vi "thrower Controller.vi"(8 "error in":errorcluster) -> ()   [LabVIEW 2020]
doc: "This VI executes continuously carrying out the current operation and responding to updates or new operations. It will often contain the timing or control code that is difficult to place directly in TeleOp. This VI generally opens all sensors and motors and isolates the rest of the robot code from knowing how the operations are carried out."
uses:
  <vilib>/Rock Robotics/WPI/Framework/Completion Status.ctl
  thrower Setpoints.ctl
  thrower Operations.ctl
  <vilib>/Rock Robotics/SystemInterfaces/DIO/FPGA_DIOPWMChannel.ctl
  <vilib>/Rock Robotics/SystemInterfaces/DIO/FPGA_DIOChannel.ctl
  <vilib>/Rock Robotics/WPI/ThirdParty/Phoenix-LabVIEW/Motor Controller/Controls/CTRE_Phoenix_MotorControl_ControlMode.ctl
  <vilib>/Rock Robotics/WPI/ThirdParty/REV Robotics/REVLib/Typedef/Spark MAX Control Type.ctl
  <vilib>/Rock Robotics/Network Tables/NT Write Boolean.vi
panel:
  in  "Interactive Values":T1
  out "Current\nCmd":string
  in  "Buttons":cluster{"Execute Cmd":bool, "Abort Cmd":bool}
  out "Command Timing":cluster{"Start Time (ms)":u32, "Iterations":i32}
  out "Status":T3
  # "Tip: It may be helpful to observe inputs and sensor values.\nYou may also want to display tuning or debugging controls."
  # "Interactive Command: You may fill in the settings for a command\nand schedule it with the Execute button. You can observe and abort\nany command while fine tuning the code for the controller."
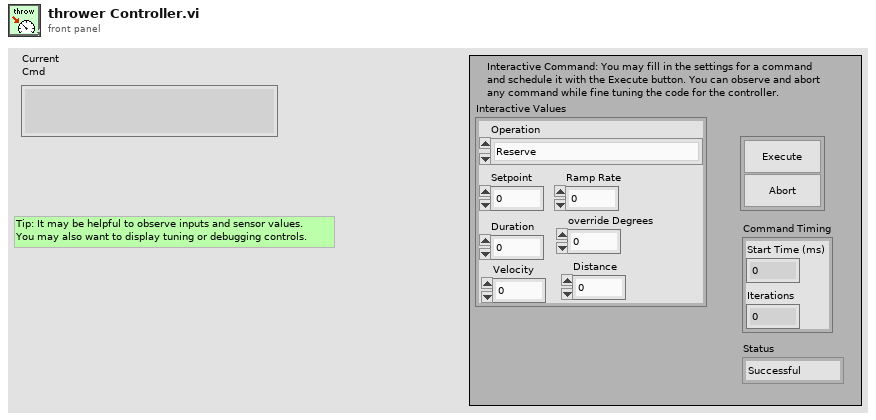
[diagram p1: front panel]
types:
  T1 = typedef "thrower Setpoints.ctl" = cluster{"Operation":T2, "Setpoint":dbl, "Duration":dbl, "Ramp Rate":dbl, "override Degrees":dbl, "Velocity":dbl, "Distance":dbl}
  T2 = typedef "thrower Operations.ctl" = enum16{"Reserve", "Read Current", "Immediate", "feed ball", "rev up thrower", "aim servos", "resetServos", "fire ball"}
  T3 = typedef "Completion Status.ctl" = enum16{"Successful", "Aborted", "Incomplete"}
  T4 = typedef "FPGA_DIOChannel.ctl" = enum8{"DIO 0", "DIO 1", "DIO 2", "DIO 3", "DIO 4", "DIO 5", "DIO 6", "DIO 7", "DIO 8", "DIO 9", "DIO MXP 0", "DIO MXP 1", "DIO MXP 2", "DIO MXP 3", "DIO MXP 4", "DIO MXP 5", "DIO MXP 6", "DIO MXP 7", "DIO MXP 8", "DIO MXP 9", "DIO MXP 10", "DIO MXP 11", "DIO MXP 12", "DIO MXP 13", "DIO MXP 14", "DIO MXP 15", "SPI Port CS1", "SPI Port CS2", "SPI Port CS3", "SPI Port MISO", "SPI Port MOSI", "Invalid"}
  T5 = typedef "FPGA_DIOPWMChannel.ctl" = enum8{"PWM 0", "PWM 1", "PWM 2", "PWM 3", "PWM 4", "PWM 5", "PWM 6", "PWM 7", "PWM 8", "PWM 9", "PWM MXP 0", "PWM MXP 1", "PWM MXP 2", "PWM MXP 3", "PWM MXP 4", "PWM MXP 5", "PWM MXP 6", "PWM MXP 7", "PWM MXP 8", "PWM MXP 9", "Invalid"}
  T6 = typedef "WPI_MotorControlDeviceRef.ctl" = cluster{"DeviceStatus":errorcluster, "Type":T7, "PWM":cluster{"PWM Channel":T5, "DeadBand":T8}, "CAN":cluster{"Device Number":u8, "SetOutput VI Ref":variant, "GetOutput VI Ref":variant, "Enable VI Ref":variant, "Disable VI Ref":variant, "Data":variant}, "Invert":bool, "DIO PWM":cluster{"PWM \"Enable\" Channel":T5, "DIOChannel":T4, "PWM Rate":dbl}}
  T7 = typedef "WPI_MotorControlType.ctl" = enum16{"PWM", "CAN", "DIO PWM"}
  T8 = typedef "WPI_PWMDeadband.ctl" = cluster{"Name":string, "maxPositivePwm":i32, "minPositivePwm":i32, "centerPwm":i32, "maxNegativePwm":i32, "minNegativePwm":i32, "angularRange":u16}
  T9 = typedef "WPI_ServoDeviceRef.ctl" = cluster{"DeviceStatus":errorcluster, "PWM Channel":T5, "DeadBand":T8}
  T10 = typedef "WPI_DigitalInputDevRef.ctl" = cluster{"DevStatus":errorcluster, "DIO Channel":T4}
  T11 = typedef "Command Status Info.ctl" = cluster{"Name":string, "Status":T3, "notifier out":T12}
  T12 = typedef "Completion Notifier.ctl" = refnum<notifier>
  T13 = cluster{"Current Command":T1, "Command Timing":cluster{"Start Time (ms)":u32, "Iterations":i32}, "Command Arguments":cluster{"Command Info":T11, "Description":string, "Default Command":T1, "queue out":refnum<queue>, "Subsystem Name":string}}
  T14 = typedef "Spark MAX Control Type.ctl" = enum16{"Percent VBus", "Voltage", "Velocity", "Position", "Smart Motion", "Current", "Smart Velocity"}
  T15 = typedef "CTRE_Phoenix_MotorControl_ControlMode.ctl" = u16
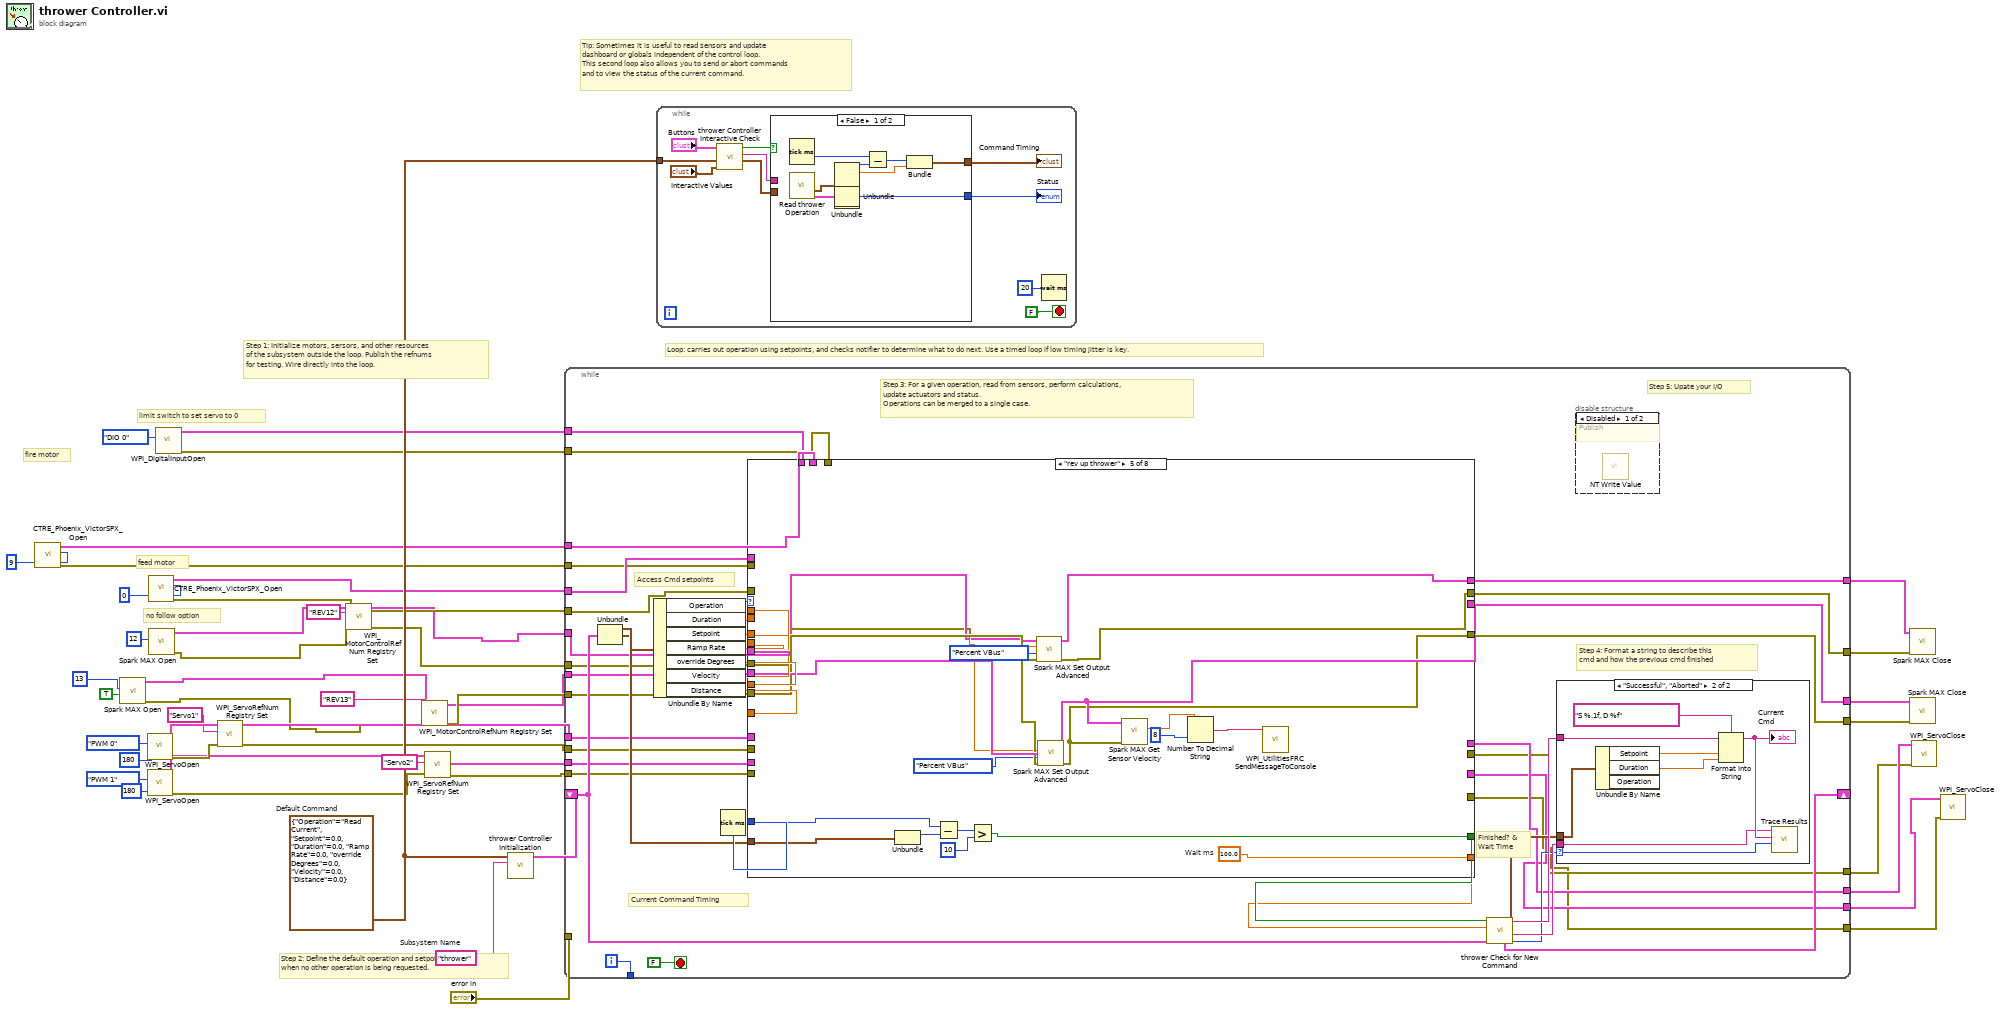
[diagram p0: block diagram]
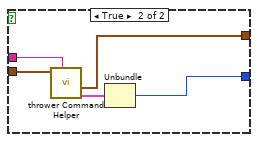
[diagram p2: hidden frame]
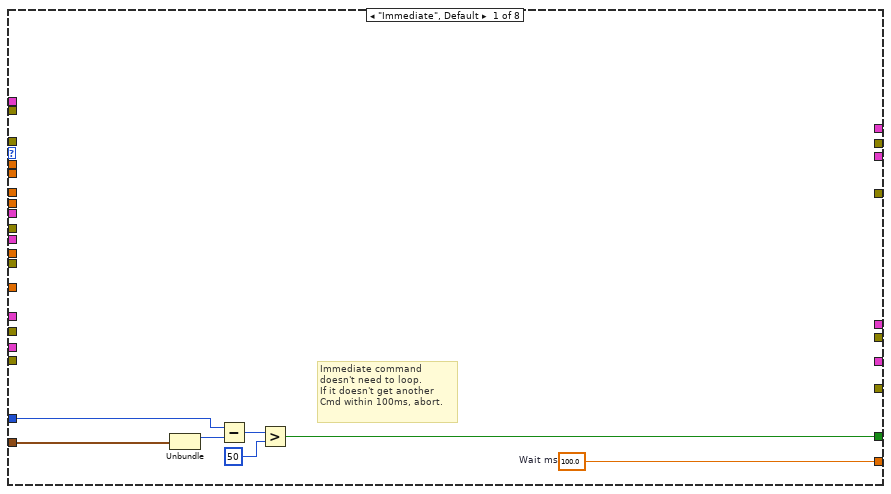
[diagram p5: hidden frame]
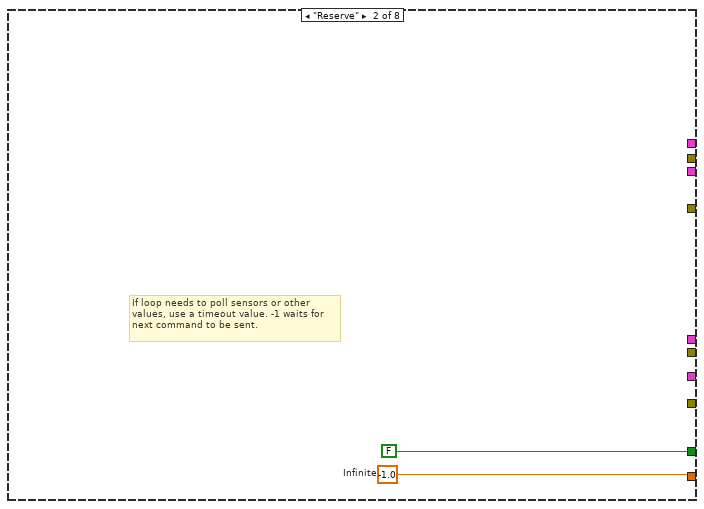
[diagram p6: hidden frame]
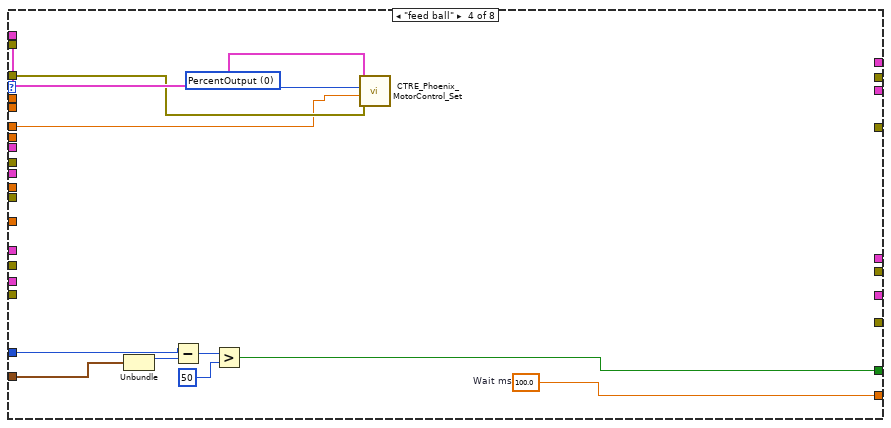
[diagram p8: hidden frame]
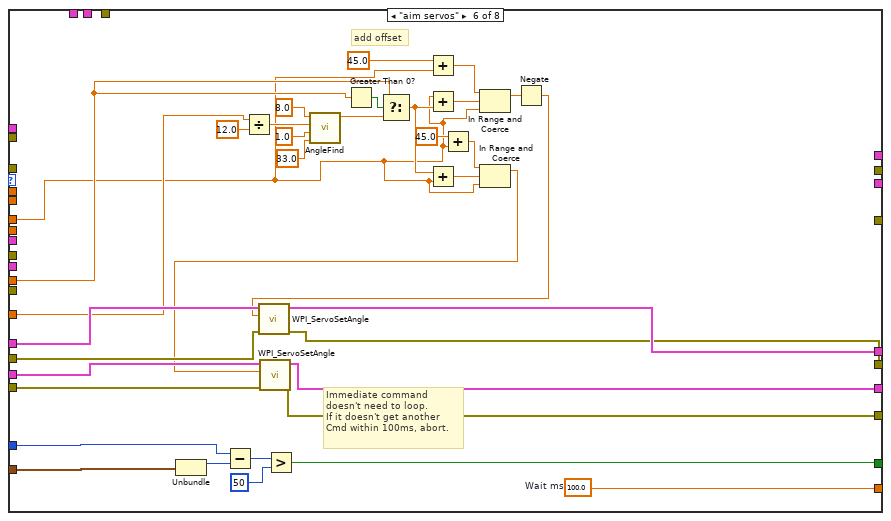
[diagram p9: hidden frame]
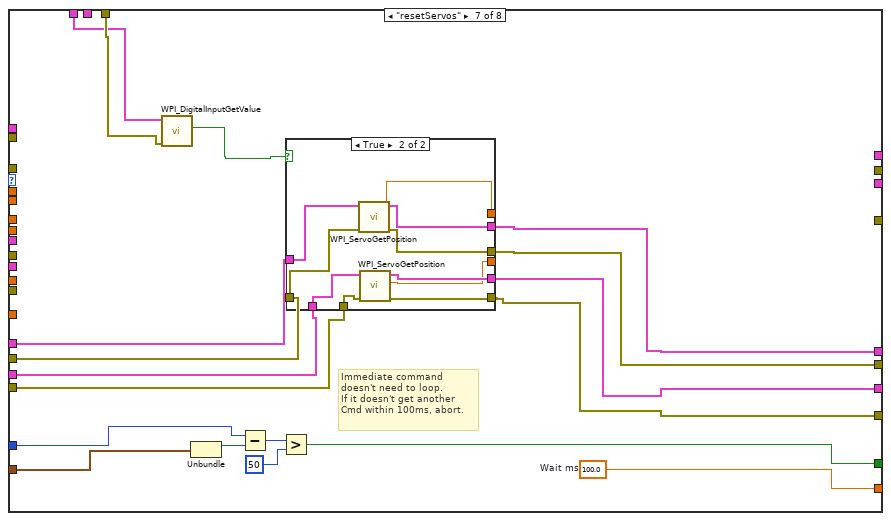
[diagram p10: hidden frame]
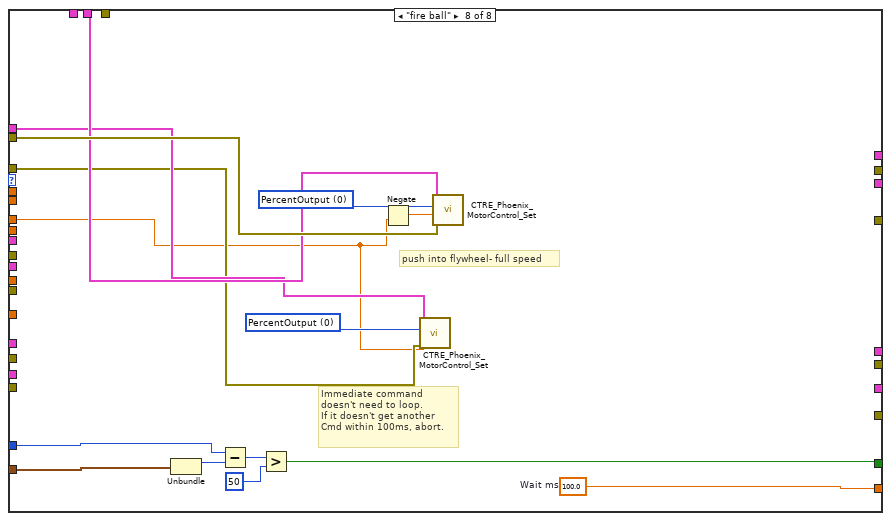
[diagram p12: hidden frame]
diagram:
  w45 = T1 {"Operation"=enum."Read Current", "Setpoint"=0.0, "Duration"=0.0, "Ramp Rate"=0.0, "override Degrees"=0.0, "Velocity"=0.0, "Distance"=0.0}  # Default Command
  w46 = "thrower"  # Subsystem Name
  # "fire motor"
  # "limit switch to set servo to 0"
  # "no follow option"
  # "feed motor"
  # "Tip: Sometimes it is useful to read sensors and update\ndashboard or globals independent of the control loop.\nThis second loop also allows you to send or abort commands\nand to view the status of the current command."
  # "Step 2: Define the default operation and setpoint --\nwhen no other operation is being requested."
  # "Step 1: Initialize motors, sersors, and other resources\nof the subsystem outside the loop. Publish the refnums\nfor testing. Wire directly into the loop."
  # "Loop: carries out operation using setpoints, and checks notifier to determine what to do next. Use a timed loop if low timing jitter is key."
  n1 = call <vilib>:"CTRE_Phoenix_VictorSPX_Open.vi"("Device Number"=u8 9) -> ("error out"=w30:errorcluster, "PhoenixMotorControlDevRef"=w31:T6)  [unwired: 9 in]
  n2 = call <vilib>:"Spark MAX Open.vi"("Invert"=TRUE, "Device Number"=u8 13) -> ("error out"=w7:errorcluster, "MotorControlDeviceRef"=w6:T6)  [unwired: 8 in]
  n3 = call <vilib>:"WPI_ServoOpen.vi"("Angular Range"=u16 180, "PWM Channel"=FPGA_DIOPWMChannel."PWM 0") -> ("error out"=w19:errorcluster, "ServoDeviceRef"=w18:T9)  [unwired: 8 in]
  n4 = call <vilib>:"WPI_ServoOpen.vi"("Angular Range"=u16 180, "PWM Channel"=FPGA_DIOPWMChannel."PWM 1") -> ("error out"=w15:errorcluster, "ServoDeviceRef"=w12:T9)  [unwired: 8 in]
  n5 = call <vilib>:"CTRE_Phoenix_VictorSPX_Open.vi"("Device Number"=u8 0) -> ("error out"=w43:errorcluster, "PhoenixMotorControlDevRef"=w44:T6)  [unwired: 9 in]
  n6 = call <vilib>:"Spark MAX Open.vi"("Device Number"=u8 12) -> ("error out"=w4:errorcluster, "MotorControlDeviceRef"=w5:T6)  [unwired: 9 in]
  n7 = call <vilib>:"WPI_DigitalInputOpen.vi"("DIO Channel"=FPGA_DIOChannel."DIO 0") -> ("error out"=w35:errorcluster, "DigitalInputDevRef"=w34:T10)  [unwired: 9 in]
  n8 = call <vilib>:"WPI_ServoRefNum Registry Set.vi"("error in (no error)"=w19, "refnum name"="Servo1", "ServoDeviceRef"=w18) -> ("error out"=w16:errorcluster, "ServoDeviceRef"=w17:T9)  [unwired: 7 in]
  n9 = call <vilib>:"WPI_MotorControlRefNum Registry Set.vi"("error in (no error)"=w4, "refnum name"="REV12", "MotorControlDevRef"=w5) -> ("error out"=w21:errorcluster, "MotorControlDevRef"=w20:T6)  [unwired: 7 in]
  n10 = call <vilib>:"WPI_MotorControlRefNum Registry Set.vi"("error in (no error)"=w7, "refnum name"="REV13", "MotorControlDevRef"=w6) -> ("error out"=w23:errorcluster, "MotorControlDevRef"=w3:T6)  [unwired: 7 in]
  n11 = call <vilib>:"WPI_ServoRefNum Registry Set.vi"("error in (no error)"=w15, "refnum name"="Servo2", "ServoDeviceRef"=w12) -> ("error out"=w14:errorcluster, "ServoDeviceRef"=w13:T9)  [unwired: 7 in]
  n12 = call "thrower Controller Initialization.vi"("Subsystem Name"=w46, "Default Command"=w45) -> ("Current Command"=w47:T13)  [unwired: 9 in]
  n13 = while {
    shift-right: [w82] -> _
    shift-left: w47 -> [w75]
    tunnel: [w89] -> _
    tunnel: "error in" -> [_]
    tunnel: w44 -> [w74]
    tunnel: w43 -> [w73]
    tunnel: w20 -> [w72]
    tunnel: w3 -> [w71]
    tunnel: w21 -> [w70]
    tunnel: w23 -> [w69]
    tunnel: w17 -> [w67]
    tunnel: w13 -> [w66]
    tunnel: w16 -> [w65]
    tunnel: w14 -> [w64]
    tunnel: [w63] -> w39
    tunnel: [w62] -> w38
    tunnel: [w61] -> w37
    tunnel: [w60] -> w36
    tunnel: w35 -> [w50]
    tunnel: w34 -> [w49]
    tunnel: w31 -> [w56]
    tunnel: w30 -> [w55]
    tunnel: [w54] -> w29
    tunnel: [w53] -> w28
    tunnel: [w52] -> w27
    tunnel: [w51] -> w26
    i -> [w89]
    stop <- FALSE stop-if-true
    # "Step 5: Upate your I/O"
    # "Step 4: Format a string to describe this\ncmd and how the previous cmd finished"
    # "Current Command Timing"
    # "Access Cmd setpoints"
    # "Finished? &\nWait Time"
    # "Step 3: For a given operation, read from sensors, perform calculations,\nupdate actuators and status.\nOperations can be merged to a single case."
    n14 = Unbundle(w75) -> ("Current Command"=w88:T1, "Command Timing"=w84:cluster{"Start Time (ms)":u32, "Iterations":i32})  [unwired: 1 out]
    n15 = Unbundle By Name(w88) -> ("Operation"=w87:T2, "Duration"=w86:dbl, "Setpoint"=w83:dbl, "Ramp Rate"=w68:dbl, "override Degrees"=w59:dbl, "Velocity"=w58:dbl, "Distance"=w57:dbl)
    n16 = Tick Count (ms)() -> (millisecond timer value=w85:u32)
    n17 = case shown="\"rev up thrower\"" w87 {
      tunnel: [w105 w107 _ w109 w137 w140 w177 w203] -> w80
      tunnel: [w99 FALSE ("ignore previous (F)") _ w110 w136 w141 w178 w204] -> w81
      tunnel: w84 -> [w101 _ _ w112 w139 w142 w179 w205]
      tunnel: w86 -> [_ _ _ _ _ _ _ _]
      tunnel: w85 -> [w100 _ _ w111 w138 w143 w180 w206]
      tunnel: w83 -> [_ _ _ w108 w131 w147 _ w210]
      tunnel: w74 -> [_ _ _ w118 _ _ _ w213]
      tunnel: w73 -> [_ _ _ w117 _ _ _ w212]
      tunnel: w72 -> [_ _ _ _ w129 _ _ _]
      tunnel: w71 -> [_ _ _ _ w135 _ _ _]
      tunnel: w70 -> [_ _ _ _ w128 _ _ _]
      tunnel: w69 -> [_ _ _ _ w134 _ _ _]
      tunnel: w68 -> [_ _ _ _ _ _ _ _]
      tunnel: w67 -> [_ _ _ _ _ w174 w191 _]
      tunnel: w66 -> [_ _ _ _ _ w173 w187 _]
      tunnel: w65 -> [_ _ _ _ _ w172 w190 _]
      tunnel: w64 -> [_ _ _ _ _ w171 w186 _]
      tunnel: [_ _ _ _ _ w170 w189 _] -> w63
      tunnel: [_ _ _ _ _ w169 w188 _] -> w62
      tunnel: [_ _ _ _ _ w168 w184 _] -> w61
      tunnel: [_ _ _ _ _ w167 w185 _] -> w60
      tunnel: w59 -> [_ _ _ _ _ w158 _ _]
      tunnel: w58 -> [_ _ _ _ _ _ _ _]
      tunnel: w57 -> [_ _ _ _ _ w157 _ _]
      tunnel: w56 -> [_ _ _ _ _ _ _ w214]
      tunnel: w55 -> [_ _ _ _ _ _ _ w215]
      tunnel: [_ _ _ _ w130 _ _ _] -> w54
      tunnel: [_ _ _ _ w127 _ _ _] -> w53
      tunnel: [_ _ _ _ w133 _ _ _] -> w52
      tunnel: [_ _ _ _ w132 _ _ _] -> w51
      tunnel: w50 -> [_ _ _ _ _ _ w176 _]
      tunnel: w49 -> [_ _ _ _ _ _ w175 _]
      frame "Immediate", Default {
        w105 = 100.0  # Wait ms
        # "Immediate command\ndoesn't need to loop.\nIf it doesn't get another\nCmd within 100ms, abort."
        n18 = Unbundle(w101) -> ("Start Time (ms)"=w104:u32)  [unwired: 1 out]
        n19 = Subtract(x=w100, y=w104) -> (x-y=w103:u32)
        n20 = Greater?(x=w103, y=u8 50 ("Left Motor")) -> (0:w99:bool)
      }
      frame "Reserve" {
        w107 = -1.0  # Infinite
        # "If loop needs to poll sensors or other\nvalues, use a timeout value. -1 waits for\nnext command to be sent."
      }
      frame "Read Current" {
      }
      frame "feed ball" {
        w109 = 100.0  # Wait ms
        w116 = T15 0 items=["PercentOutput"=0, "Position"=1, "Velocity"=2, "Current"=3, "Follower"=5, "MotionProfile"=6, "MotionMagic"=7, "MotionProfileArc"=10, "Disabled"=15] ("Control Mode")
        n21 = Unbundle(w112) -> ("Start Time (ms)"=w115:u32)  [unwired: 1 out]
        n22 = Subtract(x=w111, y=w115) -> (x-y=w114:u32)
        n23 = Greater?(x=w114, y=u8 50 ("Left Motor")) -> (0:w110:bool)
        n24 = call <vilib>:"CTRE_Phoenix_MotorControl_Set.vi"("error in (no error)"=w117, "Output"=w108, "Control Mode"=w116, "PhoenixMotorControlDevRef"=w118) -> ()  [unwired: 6 in, 2 out]
      }
      frame "rev up thrower" {
        w137 = 100.0  # Wait ms
        n25 = Unbundle(w139) -> ("Start Time (ms)"=w126:u32)  [unwired: 1 out]
        n26 = Subtract(x=w138, y=w126) -> (x-y=w125:u32)
        n27 = Greater?(x=w125, y=u8 10 ("Left Motor")) -> (0:w136:bool)
        n28 = call <vilib>:"Spark MAX Set Output Advanced.vi"("error in (no error)"=w128, "Control Mode"=Spark_MAX_Control_Type."Percent VBus", "Setpoint"=w131, "MotorControlDevRef"=w129) -> ("error out"=w127:errorcluster, "MotorControlDevRef"=w130:T6)  [unwired: 6 in]
        n29 = call <vilib>:"Spark MAX Set Output Advanced.vi"("error in (no error)"=w134, "Control Mode"=Spark_MAX_Control_Type."Percent VBus", "Setpoint"=w131, "MotorControlDevRef"=w135) -> ("error out"=w132:errorcluster, "MotorControlDevRef"=w133:T6)  [unwired: 6 in]
        n30 = call <vilib>:"Spark MAX Get Sensor Velocity.vi"("error in (no error)"=w132, "MotorControlDevRef in"=w133) -> ("Sensor Velocity"=w123:dbl)  [unwired: 6 in, 3 out]
        n31 = Number To Decimal String(number=w123, width (-)=i16 8) -> (decimal integer string=w121:string)
        n32 = call <vilib>:"WPI_UtilitiesFRC SendMessageToConsole.vi"("Message"=w121) -> ()  [unwired: 14 in, 1 out]
      }
      frame "aim servos" {
        w140 = 100.0  # Wait ms
        # "Immediate command\ndoesn't need to loop.\nIf it doesn't get another\nCmd within 100ms, abort."
        # "add offset"
        n33 = Unbundle(w142) -> ("Start Time (ms)"=w146:u32)  [unwired: 1 out]
        n34 = Subtract(x=w143, y=w146) -> (x-y=w145:u32)
        n35 = Divide(x=w157, y=12.0) -> (x/y=w161:dbl)
        n36 = Greater?(x=w145, y=u8 50 ("Left Motor")) -> (0:w141:bool)
        n37 = call "AngleFind.vi"("Speed Sent (ft)"=33.0, "Distance off Ground (ft)"=1.0, "Distance to Target (Ground Distance) (ft)"=w161, "Height of Target (ft)"=8.0) -> ("Angle (Degrees?)"=w159:dbl)  [unwired: 7 in]
        n38 = Greater Than 0?(x=w158) -> (x > 0?=w160:bool)
        n39 = Select(t=w158, s=w160, f=w159) -> (s? t:f=w156:dbl)
        n40 = Add(x=45.0, y=w147) -> (x+y=w151:dbl)
        n41 = Add(x=w147, y=w156) -> (x+y=w152:dbl)
        n42 = Add(x=w156, y=w147) -> (x+y=w153:dbl)
        n43 = Add(x=45.0, y=w147) -> (x+y=w148:dbl)
        n44 = In Range and Coerce(upper limit=w151, x=w152, lower limit=w147) -> (coerced(x)=w155:dbl)  [unwired: 1 out]
        n45 = In Range and Coerce(upper limit=w148, x=w153, lower limit=w147) -> (coerced(x)=w154:dbl)  [unwired: 1 out]
        n46 = call <vilib>:"WPI_ServoSetAngle.vi"("error in (no error)"=w171, "Angle"=w154, "ServoDeviceRef"=w173) -> ("error out"=w167:errorcluster, "ServoDeviceRef"=w168:T9)  [unwired: 7 in]
        n47 = Negate(x=w155) -> (-x=w166:dbl)
        n48 = call <vilib>:"WPI_ServoSetAngle.vi"("error in (no error)"=w172, "Angle"=w166, "ServoDeviceRef"=w174) -> ("error out"=w169:errorcluster, "ServoDeviceRef"=w170:T9)  [unwired: 7 in]
      }
      frame "resetServos" {
        w177 = 100.0  # Wait ms
        # "Immediate command\ndoesn't need to loop.\nIf it doesn't get another\nCmd within 100ms, abort."
        n49 = call <vilib>:"WPI_DigitalInputGetValue.vi"("error in (no error)"=w176, "DigitalInputDevRef"=w175) -> ("Value"=w192:bool)  [unwired: 7 in, 2 out]
        n50 = Unbundle(w179) -> ("Start Time (ms)"=w183:u32)  [unwired: 1 out]
        n51 = Subtract(x=w180, y=w183) -> (x-y=w182:u32)
        n52 = Greater?(x=w182, y=u8 50 ("Left Motor")) -> (0:w178:bool)
        n53 = case shown="True" w192 {
          tunnel: w191 -> [_ w202]
          tunnel: w190 -> [_ w201]
          tunnel: [_ w200] -> w189
          tunnel: [_ w199] -> w188
          tunnel: w187 -> [_ w198]
          tunnel: w186 -> [_ w197]
          tunnel: [_ w196] -> w185
          tunnel: [_ w195] -> w184
          tunnel: [_ w194] -> _
          tunnel: [_ w193] -> _
          frame False {
          }
          frame True {
            n54 = call <vilib>:"WPI_ServoGetPosition.vi"("error in (no error)"=w201, "ServoDeviceRef"=w202) -> ("error out"=w199:errorcluster, "Position"=w194:dbl, "ServoDeviceRef"=w200:T9)  [unwired: 7 in]
            n55 = call <vilib>:"WPI_ServoGetPosition.vi"("error in (no error)"=w197, "ServoDeviceRef"=w198) -> ("error out"=w196:errorcluster, "Position"=w193:dbl, "ServoDeviceRef"=w195:T9)  [unwired: 7 in]
          }
        }
      }
      frame "fire ball" {
        w203 = 100.0  # Wait ms
        w216 = T15 0 items=["PercentOutput"=0, "Position"=1, "Velocity"=2, "Current"=3, "Follower"=5, "MotionProfile"=6, "MotionMagic"=7, "MotionProfileArc"=10, "Disabled"=15] ("Control Mode")
        w217 = T15 0 items=["PercentOutput"=0, "Position"=1, "Velocity"=2, "Current"=3, "Follower"=5, "MotionProfile"=6, "MotionMagic"=7, "MotionProfileArc"=10, "Disabled"=15] ("Control Mode")
        # "Immediate command\ndoesn't need to loop.\nIf it doesn't get another\nCmd within 100ms, abort."
        # "push into flywheel- full speed"
        n56 = Unbundle(w205) -> ("Start Time (ms)"=w208:u32)  [unwired: 1 out]
        n57 = Subtract(x=w206, y=w208) -> (x-y=w209:u32)
        n58 = Greater?(x=w209, y=u8 50 ("Left Motor")) -> (0:w204:bool)
        n59 = Negate(x=w210) -> (-x=w211:dbl)
        n60 = call <vilib>:"CTRE_Phoenix_MotorControl_Set.vi"("error in (no error)"=w212, "Output"=w210, "Control Mode"=w216, "PhoenixMotorControlDevRef"=w213) -> ()  [unwired: 6 in, 2 out]
        n61 = call <vilib>:"CTRE_Phoenix_MotorControl_Set.vi"("error in (no error)"=w215, "Output"=w211, "Control Mode"=w217, "PhoenixMotorControlDevRef"=w214) -> ()  [unwired: 6 in, 2 out]
      }
    }
    n62 = call "thrower Check for New Command.vi"("Current Command"=w75, "Wait time (ms)"=w80, "Finished?"=w81) -> ("Completion"=w76:T3, "Subsystem Name"=w77:string, "Current Command"=w78:T1, "Initial Trace String"=w79:string, "NextCommand"=w82:T13)  [unwired: 4 in]
    n63 = case shown="\"Successful\", \"Aborted\"" w76 {
      selector: w76 -> [_ w98]
      tunnel: w79 -> [_ w94]
      tunnel: w78 -> [_ w95]
      tunnel: w77 -> [_ w91]
      frame "Incomplete", Default {
        # "Continuing current command"
      }
      frame "Successful", "Aborted" {
        # "Report and setup for next command"
        n64 = Unbundle By Name(w95) -> ("Setpoint"=w97:dbl, "Duration"=w92:dbl)  [unwired: 1 out]
        n65 = Format Into String(format string="S %.1f, D %f", initial string=w94, w97, w92) -> (resulting string=w93:string)  [unwired: 1 in, 1 out]
        "Current\nCmd" <- w93
        n66 = call <vilib>:"Trace Results.vi"("Status of previous command"=w98, "Description"=w93, "Subsystem"=w91) -> ()  [unwired: 9 in]
      }
    }
    n67 = disable-structure shown="Disabled" {
      frame Disabled {
        # "Publish"
        n68 = call-poly <vilib>:"NT Write Value.vi"() -> ()  [unwired: 11 in, 1 out]
      }
      frame Enabled {
      }
    }
  }
  n69 = while {
    tunnel: w45 -> [w218]
    stop <- FALSE stop-if-true
    n70 = call "thrower Controller Interactive Check.vi"("Interactive Command in"="Interactive Values", "Default Command"=w218, "Buttons"="Buttons") -> ("Interactive Command out"=w222:T1, "Trace String"=w223:string, "Schedule"=w224:bool)  [unwired: 6 in]
    n71 = case shown="False" w224 {
      tunnel: [w235 w240] -> w221
      tunnel: w222 -> [_ w238]
      tunnel: [w231 w236] -> w220
      tunnel: w223 -> [_ w239]
      frame False {
        n72 = Tick Count (ms)() -> (millisecond timer value=w230:u32)
        n73 = call "Read thrower Operation.vi"() -> ("Command Info"=w228:T11, "SubSystem Data"=w229:T1)  [unwired: 9 in, 1 out]
        n74 = Unbundle(w229) -> ("Operation"=w234:T2, "Setpoint"=w232:dbl)  [unwired: 5 out]
        n75 = Unbundle(w228) -> ("Status"=w235:T3)  [unwired: 2 out]
        n76 = Subtract(x=w230, y=w234) -> (x-y=w233:u32)
        n77 = Bundle(w233, "Setpoint"=w232) -> (w231:cluster{u32, "Setpoint":dbl})  [unwired: 1 in]
      }
      frame True {
        n78 = call "thrower Command Helper.vi"("Description"=w239, "SubSystem Data"=w238) -> ("Command Info Out"=w237:T11, "Command Timing"=w236:cluster{"Start Time (ms)":u32, "Iterations":i32})  [unwired: 7 in, 1 out]
        n79 = Unbundle(w237) -> ("Status"=w240:T3)  [unwired: 2 out]
      }
    }
    "Status" <- w221
    "Command Timing" <- w220
    n80 = Wait (ms)(milliseconds to wait=u32 20) -> ()  [unwired: 1 out]
  }
  n81 = call <vilib>:"Spark MAX Close.vi"("error in"=w28, "MotorControlDeviceRef"=w29) -> ()  [unwired: 9 in, 1 out]
  n82 = call <vilib>:"Spark MAX Close.vi"("error in"=w26, "MotorControlDeviceRef"=w27) -> ()  [unwired: 9 in, 1 out]
  n83 = call <vilib>:"WPI_ServoClose.vi"("error in (no error)"=w38, "ServoDeviceRef"=w39) -> ()  [unwired: 9 in, 1 out]
  n84 = call <vilib>:"WPI_ServoClose.vi"("error in (no error)"=w36, "ServoDeviceRef"=w37) -> ()  [unwired: 9 in, 1 out]
